vi "Set Live img window UI from file-Boolean.vi"(8 "error in (no error)":errorcluster, 9 "Keys setup.Boolean":T2, 10 "Section name":string, 11 "Refnum in":T1) -> (0 "error out":errorcluster, 3 "Refnum out":T1)   [LabVIEW 2017]
uses:
  Typedefs/Ini file interface (Boolean).ctl
  <vilib>/Utility/config.llb/Config Data RefNum.ctl
  User Interface/Globals/gl_Windows Ctrl refs.vi
  <vilib>/Utility/config.llb/NI_LVConfig.lvlib
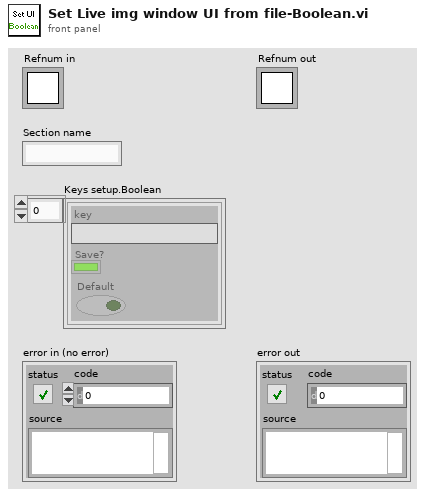
[diagram p1: front panel]
types:
  T1 = typedef "NI_LVConfig.lvlib/Config Data RefNum.ctl" = refnum<k1>
  T2 = typedef "Ini file interface (Boolean).ctl" = cluster{"key":string, "Save?":bool, "Default":bool}[]
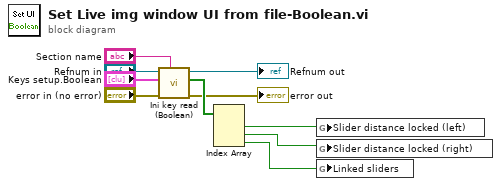
[diagram p0: block diagram]
diagram:
  n1 = call "Ini key read (Boolean).vi"("Section"="Section name", "error in (no error)"="error in (no error)", "Parameter names & setup"="Keys setup.Boolean", "Ini file refnum in"="Refnum in") -> ("error out"=→"error out":errorcluster, "Value read/used"=w10:bool[], "Ini file refnum out"=→"Refnum out":T1)  [unwired: 5 in]
  n2 = Index Array(array=w10) -> (element #1=w3:bool, element #2=w2:bool, element #3=w1:bool)  [unwired: 3 in]
  n3 = global write "gl_Windows Ctrl refs.vi" "Slider distance locked (left)"(w3) -> ()
  n4 = global write "gl_Windows Ctrl refs.vi" "Slider distance locked (right)"(w2) -> ()
  n5 = global write "gl_Windows Ctrl refs.vi" "Linked sliders"(w1) -> ()
